vi "initialise channel scaling.vi"() -> ()   [LabVIEW 2018]
uses:
  PC/type defs/channelControl.ctl
  Type Defs/channelScalingTypes.ctl
  Type Defs/scalingMethods.ctl
panel:
  out "channelScales":T1[](array[typedef])
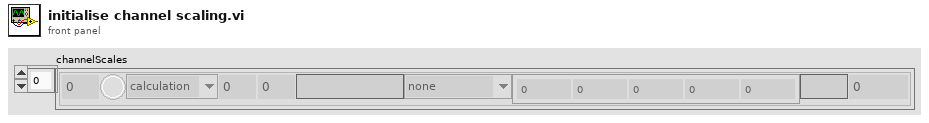
[diagram p1: front panel]
types:
  T1 = typedef "channelControl.ctl" = cluster{"index":u16, "active":bool, "channelType":T2, "module":u16, "terminal":u16, "channelName":string, "scalingMethod":T3, "scalingParameters":dbl[], "scaledUnits":string, "tempOffset":dbl}
  T2 = typedef "channelScalingTypes.ctl" = enum16{"calculation", "measurement", "scanivalve", "output", "digital"}
  T3 = typedef "scalingMethods.ctl" = enum16{"none", "linear", "thermocouple", "polynomial", "encoder", "RTD"}
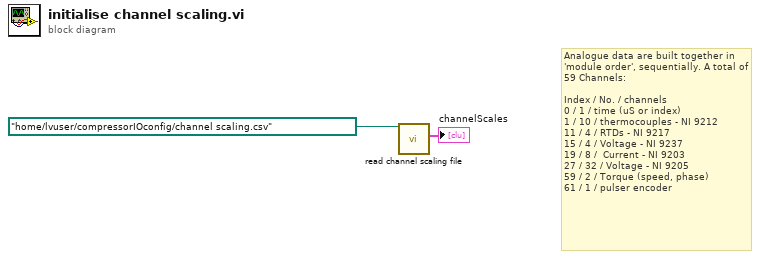
[diagram p0: block diagram]
diagram:
  # "Analogue data are built together in 'module order', sequentially. A total of 59 Channels:\n\nIndex / No. / channels\n0 / 1 / time (uS or index)\n1 / 10 / thermocouples - NI 9212\n11 / 4 / RTDs - NI 9217\n15 / 4 / Voltage - NI 9237\n19 / 8 /  Current - NI 9203\n27 / 32 / Voltage - NI 9205\n59 / 2 / Torque (speed, phase)\n61 / 1 / pulser encoder"
  n1 = call "read channel scaling file.vi"("file path"=path "/home/lvuser/compressorIOconfig/channel scaling.csv" ("file path (use dialog)")) -> ("channelConfig"=→"channelScales":T1[])  [unwired: 6 in, 4 out]
